vi "Initialize Instrument.vi"(8 "error in (no error)":errorcluster, 10 "Reset":bool, 11 "VNA-PNA in":refnum<class "VNA-PNA.lvclass">) -> (0 "error out":errorcluster, 3 "VNA-PNA out":refnum<class "VNA-PNA.lvclass">)   [LabVIEW 2020, in "VNA-PNA.lvclass"]
uses:
  VNA-PNA.lvclass
  C:/Sandbox/RF Bench/Source Code/WiSpry Test Framework/Instruments/Instrument.lvclass
  C:/Sandbox/RF Bench/Source Code/WiSpry Test Framework/Instruments/Vector Network Analyzer/Vector Network Analyzer.lvclass
  <vilib>/Instr/_visa.llb/VISA Open Access Mode.ctl
  Instrument.lvclass/Instrument.ctl
  Vector Network Analyzer.lvclass/Vector Network Analyzer.ctl
  Instrument.lvclass
  Vector Network Analyzer.lvclass
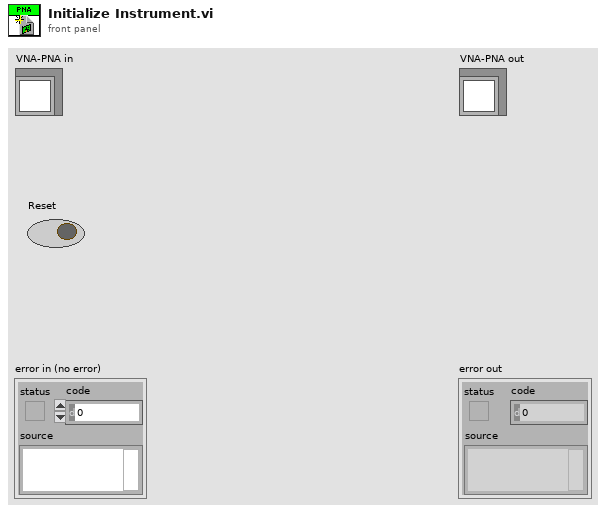
[diagram p1: front panel]
types:
  T1 = typedef "VISA Open Access Mode.ctl" = u32
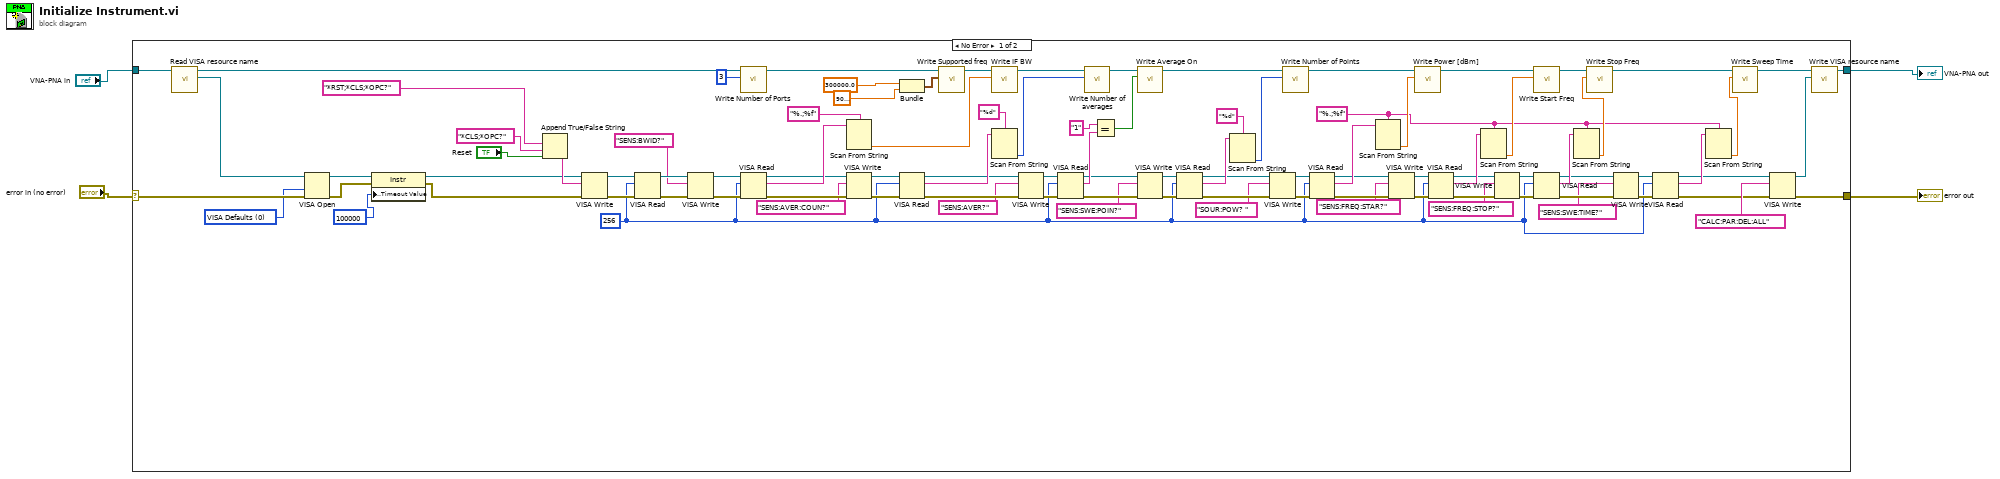
[diagram p0: block diagram]
diagram:
  n1 = case shown="No Error" "error in (no error)" {
    selector: "error in (no error)" -> [w101 w103]
    tunnel: "VNA-PNA in" -> [w102 w104]
    tunnel: [w7 w103] -> w2
    tunnel: [w68 w104] -> w1
    frame No Error {
      w11 = "%.;%f" ("format string")
      w15 = u32 256 ("byte count")
      w99 = T1 0 items=["VISA Defaults"=0, "Exclusive Lock"=1, "Load Configured Settings"=4] ("Access Mode")
      n2 = call "Read VISA resource name.vi"("Instrument in"=w102) -> ("VISA resource name"=w100:refnum<visa-resource-name>, "Instrument out"=w95:refnum<class "VNA-PNA.lvclass">)  [unwired: 9 in]
      n3 = VISA Open(access mode=w99, error in (no error)=w101, VISA resource name=w100) -> (VISA resource name=w97:refnum<visa-resource-name>, error out=w96:errorcluster)  [unwired: 2 in]
      n4 = property class="Instr"(reference=w97, error in=w96, "General Settings:Timeout Value"=u32 100000) -> (reference out=w22:refnum<visa-resource-name>, error out=w21:errorcluster)
      n5 = Append True/False String(1:"Reset", 2:"*CLS;*OPC?" ("false string"), 3:"*RST;*CLS;*OPC?" ("Default Setup String")) -> (0:w92:string)  [unwired: 1 in]
      n6 = VISA Write(VISA resource name=w22, write buffer=w92, error in (no error)=w21) -> (VISA resource name out=w90:refnum<visa-resource-name>, error out=w91:errorcluster)  [unwired: 1 out]
      n7 = VISA Read(VISA resource name=w90, byte count=w15, error in (no error)=w91) -> (VISA resource name out=w75:refnum<visa-resource-name>, error out=w76:errorcluster)  [unwired: 2 out]
      n8 = VISA Write(VISA resource name=w75, write buffer="SENS:BWID?", error in (no error)=w76) -> (VISA resource name out=w77:refnum<visa-resource-name>, error out=w73:errorcluster)  [unwired: 1 out]
      n9 = call "Write Number of Ports.vi"("Number of Ports"=3, "Vector Network Analyzer in"=w95) -> ("Vector Network Analyzer out"=w89:refnum<class "VNA-PNA.lvclass">)  [unwired: 9 in]
      n10 = VISA Read(VISA resource name=w77, byte count=w15, error in (no error)=w73) -> (VISA resource name out=w66:refnum<visa-resource-name>, read buffer=w71:string, error out=w65:errorcluster)  [unwired: 1 out]
      n11 = Scan From String(format string="%.;%f", input string=w71) -> (output 1=w70:dbl)  [unwired: 3 in, 3 out]
      n12 = VISA Write(VISA resource name=w66, write buffer="SENS:AVER:COUN?", error in (no error)=w65) -> (VISA resource name out=w63:refnum<visa-resource-name>, error out=w67:errorcluster)  [unwired: 1 out]
      n13 = Bundle(300000.0, 9000000000.0) -> (w88:cluster{dbl, dbl})  [unwired: 1 in]
      n14 = VISA Read(VISA resource name=w63, byte count=w15, error in (no error)=w67) -> (VISA resource name out=w57:refnum<visa-resource-name>, read buffer=w62:string, error out=w56:errorcluster)  [unwired: 1 out]
      n15 = call "Write Supported freq.vi"("Supported freq"=w88, "Vector Network Analyzer in"=w89) -> ("Vector Network Analyzer out"=w69:refnum<class "VNA-PNA.lvclass">)  [unwired: 9 in]
      n16 = call "Write IF BW.vi"("IF BW"=w70, "Vector Network Analyzer in"=w69) -> ("Vector Network Analyzer out"=w87:refnum<class "VNA-PNA.lvclass">)  [unwired: 9 in]
      n17 = Scan From String(format string="%d", input string=w62) -> (output 1=w60:i32)  [unwired: 3 in, 3 out]
      n18 = VISA Write(VISA resource name=w57, write buffer="SENS:AVER?", error in (no error)=w56) -> (VISA resource name out=w59:refnum<visa-resource-name>, error out=w58:errorcluster)  [unwired: 1 out]
      n19 = VISA Read(VISA resource name=w59, byte count=w15, error in (no error)=w58) -> (VISA resource name out=w49:refnum<visa-resource-name>, read buffer=w54:string, error out=w48:errorcluster)  [unwired: 1 out]
      n20 = call "Write Number of averages.vi"("Number of averages"=w60, "Vector Network Analyzer in"=w87) -> ("Vector Network Analyzer out"=w86:refnum<class "VNA-PNA.lvclass">)  [unwired: 9 in]
      n21 = Equal?(x="1", y=w54) -> (x = y?=w52:bool)
      n22 = call "Write Average On.vi"("Average On"=w52, "Vector Network Analyzer in"=w86) -> ("Vector Network Analyzer out"=w85:refnum<class "VNA-PNA.lvclass">)  [unwired: 9 in]
      n23 = VISA Write(VISA resource name=w49, write buffer="SENS:SWE:POIN?", error in (no error)=w48) -> (VISA resource name out=w50:refnum<visa-resource-name>, error out=w51:errorcluster)  [unwired: 1 out]
      n24 = VISA Read(VISA resource name=w50, byte count=w15, error in (no error)=w51) -> (VISA resource name out=w41:refnum<visa-resource-name>, read buffer=w45:string, error out=w40:errorcluster)  [unwired: 1 out]
      n25 = Scan From String(format string="%d", input string=w45) -> (output 1=w44:i32)  [unwired: 3 in, 3 out]
      n26 = VISA Write(VISA resource name=w41, write buffer="SOUR:POW? ", error in (no error)=w40) -> (VISA resource name out=w43:refnum<visa-resource-name>, error out=w42:errorcluster)  [unwired: 1 out]
      n27 = call "Write Number of Points.vi"("Number of Points"=w44, "Vector Network Analyzer in"=w85) -> ("Vector Network Analyzer out"=w84:refnum<class "VNA-PNA.lvclass">)  [unwired: 9 in]
      n28 = VISA Read(VISA resource name=w43, byte count=w15, error in (no error)=w42) -> (VISA resource name out=w34:refnum<visa-resource-name>, read buffer=w38:string, error out=w33:errorcluster)  [unwired: 1 out]
      n29 = Scan From String(format string=w11, input string=w38) -> (output 1=w37:dbl)  [unwired: 3 in, 3 out]
      n30 = VISA Write(VISA resource name=w34, write buffer="SENS:FREQ:STAR?", error in (no error)=w33) -> (VISA resource name out=w35:refnum<visa-resource-name>, error out=w36:errorcluster)  [unwired: 1 out]
      n31 = call "Write Power [dBm].vi"("Power [dBm]"=w37, "Vector Network Analyzer in"=w84) -> ("Vector Network Analyzer out"=w83:refnum<class "VNA-PNA.lvclass">)  [unwired: 9 in]
      n32 = VISA Read(VISA resource name=w35, byte count=w15, error in (no error)=w36) -> (VISA resource name out=w28:refnum<visa-resource-name>, read buffer=w31:string, error out=w27:errorcluster)  [unwired: 1 out]
      n33 = Scan From String(format string=w11, input string=w31) -> (output 1=w30:dbl)  [unwired: 3 in, 3 out]
      n34 = VISA Write(VISA resource name=w28, write buffer="SENS:FREQ:STOP?", error in (no error)=w27) -> (VISA resource name out=w29:refnum<visa-resource-name>, error out=w25:errorcluster)  [unwired: 1 out]
      n35 = call "Write Start Freq.vi"("Start Freq"=w30, "Vector Network Analyzer in"=w83) -> ("Vector Network Analyzer out"=w82:refnum<class "VNA-PNA.lvclass">)  [unwired: 9 in]
      n36 = VISA Read(VISA resource name=w29, byte count=w15, error in (no error)=w25) -> (VISA resource name out=w18:refnum<visa-resource-name>, read buffer=w23:string, error out=w17:errorcluster)  [unwired: 1 out]
      n37 = Scan From String(format string=w11, input string=w23) -> (output 1=w24:dbl)  [unwired: 3 in, 3 out]
      n38 = call "Write Stop Freq.vi"("Stop Freq"=w24, "Vector Network Analyzer in"=w82) -> ("Vector Network Analyzer out"=w14:refnum<class "VNA-PNA.lvclass">)  [unwired: 9 in]
      n39 = VISA Write(VISA resource name=w18, write buffer="SENS:SWE:TIME?", error in (no error)=w17) -> (VISA resource name out=w19:refnum<visa-resource-name>, error out=w20:errorcluster)  [unwired: 1 out]
      n40 = VISA Read(VISA resource name=w19, byte count=w15, error in (no error)=w20) -> (VISA resource name out=w6:refnum<visa-resource-name>, read buffer=w12:string, error out=w8:errorcluster)  [unwired: 1 out]
      n41 = Scan From String(format string=w11, input string=w12) -> (output 1=w10:dbl)  [unwired: 3 in, 3 out]
      n42 = call "Write Sweep Time.vi"("Sweep Time"=w10, "Vector Network Analyzer in"=w14) -> ("Vector Network Analyzer out"=w13:refnum<class "VNA-PNA.lvclass">)  [unwired: 9 in]
      n43 = VISA Write(VISA resource name=w6, write buffer="CALC:PAR:DEL:ALL", error in (no error)=w8) -> (VISA resource name out=w5:refnum<visa-resource-name>, error out=w7:errorcluster)  [unwired: 1 out]
      n44 = call "Write VISA resource name.vi"("VISA resource name"=w5, "Instrument in"=w13) -> ("Instrument out"=w68:refnum<class "VNA-PNA.lvclass">)  [unwired: 9 in]
    }
    frame Error {
    }
  }
  "error out" <- w2
  "VNA-PNA out" <- w1
